vi "OPC (SubVI).vi"(8 "error in (no error)":errorcluster, 11 "VISA Refnum in":refnum<visa-resource-name>) -> (0 "error out":errorcluster, 3 "VISA Refnum out":refnum<visa-resource-name>)   [LabVIEW 2017]
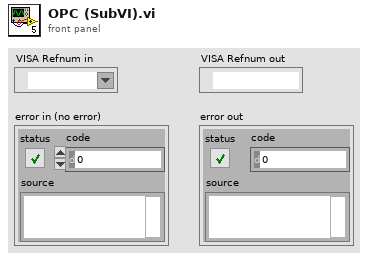
[diagram p1: front panel]
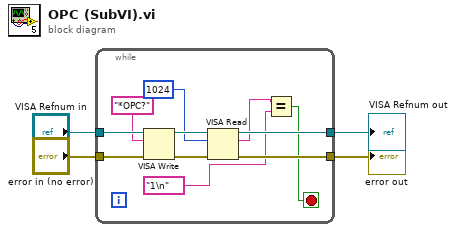
[diagram p0: block diagram]
diagram:
  n1 = while {
    tunnel: "VISA Refnum in" -> [w15]
    tunnel: "error in (no error)" -> [w14]
    tunnel: [w10] -> w3
    tunnel: [w12] -> w4
    stop <- w6 stop-if-true
    n2 = VISA Write(VISA resource name=w15, write buffer="*OPC?" ("string"), error in (no error)=w14) -> (VISA resource name out=w13:refnum<visa-resource-name>, error out=w11:errorcluster)  [unwired: 1 out]
    n3 = VISA Read(VISA resource name=w13, byte count=u32 1024, error in (no error)=w11) -> (VISA resource name out=w12:refnum<visa-resource-name>, read buffer=w8:string, error out=w10:errorcluster)  [unwired: 1 out]
    n4 = Equal?(x=w8, y="1\n" ("read buffer 3")) -> (x = y?=w6:bool)
  }
  "VISA Refnum out" <- w4
  "error out" <- w3
